vi "SetupZSpan.vi"(8 "error in (no error)":errorcluster, 10 "Center Freq (Hz)":dbl=13250000000.0 format="%#.6g", 11 "SpecA_ESA in":refnum<class "SpecA_ESA.lvclass">) -> (0 "error out":errorcluster, 3 "SpecA_ESA out":refnum<class "SpecA_ESA.lvclass">)   [LabVIEW 2014, in "SpecA_ESA.lvclass"]
uses:
  SpecA_ESA.lvclass
  SpecA_ESA.lvclass/SpecA_ESA.ctl
  data/Agilent ESA PSA Series/Configure Frequency (Center Span).vi
  data/Agilent ESA PSA Series.lvlib
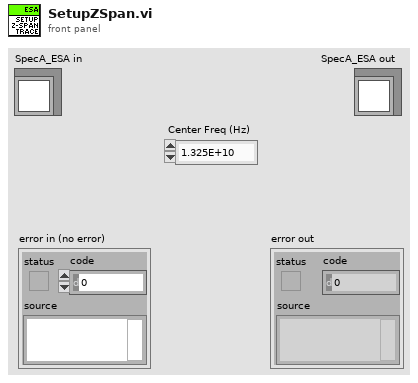
[diagram p1: front panel]
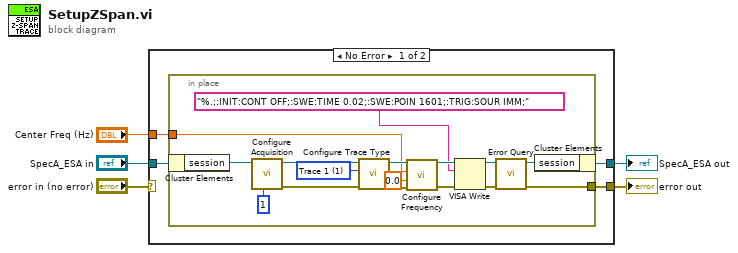
[diagram p0: block diagram]
diagram:
  n1 = case shown="No Error" "error in (no error)" {
    selector: "error in (no error)" -> [_ w27]
    tunnel: "SpecA_ESA in" -> [w9 w26]
    tunnel: [w8 w26] -> w4
    tunnel: [w7 w27] -> w2
    tunnel: "Center Freq (Hz)" -> [w6 _]
    frame No Error {
      n2 = in-place {
        in-place-border: [w19] -> w7
        in-place-border: w6 -> [w15]
        w24 = u16 1 items=["Trace 1"=1, "Trace 2"=2, "Trace 3"=3] ("Trace Name (1: Trace 1)")
        n3 = in-place-cluster #1(w9) -> ("session"=w23:refnum<visa-resource-name>)
        n4 = call "Configure Acquisition.vi"("Vertical Scale (0: Linear)"=1, "VISA resource name"=w23) -> ("error out"=w20:errorcluster, "VISA resource name out"=w21:refnum<visa-resource-name>)  [unwired: 8 in]
        n5 = call "Configure Trace Type.vi"("error in (no error)"=w20, "Trace Name (1: Trace 1)"=w24, "VISA resource name"=w21) -> ("error out"=w17:errorcluster, "VISA resource name out"=w18:refnum<visa-resource-name>)  [unwired: 7 in]
        n6 = call-poly "Configure Frequency.vi"("error in (no error)"=w17, "Span (2 GHz)"=0.0, "Center Frequency (2 GHz)"=w15, "VISA resource name"=w18) -> ("error out"=w13:errorcluster, "VISA resource name out"=w11:refnum<visa-resource-name>)  [unwired: 6 in]
        n7 = VISA Write(VISA resource name=w11, write buffer="%.;:INIT:CONT OFF;:SWE:TIME 0.02;:SWE:POIN 1601;:TRIG:SOUR IMM;" ("format string"), error in (no error)=w13) -> (VISA resource name out=w12:refnum<visa-resource-name>, error out=w14:errorcluster)  [unwired: 1 out]
        n8 = call "Error Query.vi"("error in (no error)"=w14, "VISA resource name"=w12) -> ("error out"=w19:errorcluster, "VISA resource name out"=w22:refnum<visa-resource-name>)  [unwired: 6 in, 2 out]
        n9 = in-place-cluster #1("session"=w22) -> (w8:refnum<class "SpecA_ESA.lvclass">)
      }
    }
    frame Error {
    }
  }
  "SpecA_ESA out" <- w4
  "error out" <- w2
